vi "zmq_poll.vi"   [LabVIEW 2025, in "ZeroMQ.lvlib" / "Socket.lvclass"]
uses:
  Socket.lvclass
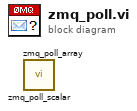
[diagram p0: block diagram]
diagram:
  n1 = call "zmq_poll_scalar.vi"() -> ()  [unwired: 4 in, 4 out]
  n2 = call "zmq_poll_array.vi"() -> ()  [unwired: 4 in, 4 out]
